vi "Update Value.vi"(6 "Time":dbl, 8 "error in (no error)":errorcluster, 11 "DblPopupControl in":refnum<class "DblPopupControl.lvclass">) -> (0 "error out":errorcluster, 1 "Update":bool, 2 "Value":variant, 3 "DblPopupControl out":refnum<class "DblPopupControl.lvclass">)   [LabVIEW 2020, in "VolatusGUIElements.lvlib" / "DblPopupControl.lvclass"]
uses:
  DblPopupControl.lvclass
  DblPopupControl.lvclass/DblPopupControl.ctl
  lv-vecto/Vecto/Channel DBL/Channel DBL.lvclass/Channel DBL.ctl
  lv-vecto/Vecto/Group DBL/Value by Index.vi
  lv-vecto/Vecto/Channel DBL/Channel DBL.lvclass
  VolatusGUIElements.lvlib
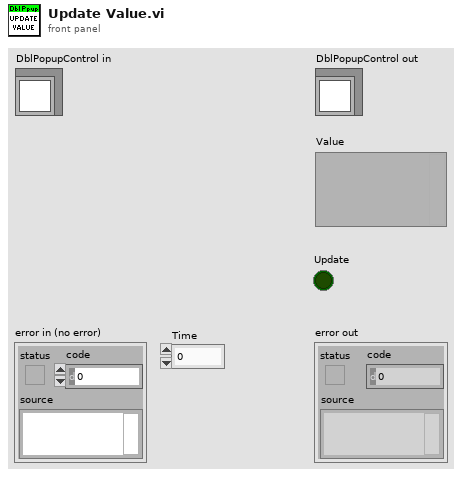
[diagram p1: front panel]
types:
  T1 = typedef "VolatusGUIElements.lvlib/DblPopupControl.lvclass/Cmd State.ctl" = cluster{"Commanding":bool, "Start":dbl, "Error":bool, "Value":dbl}
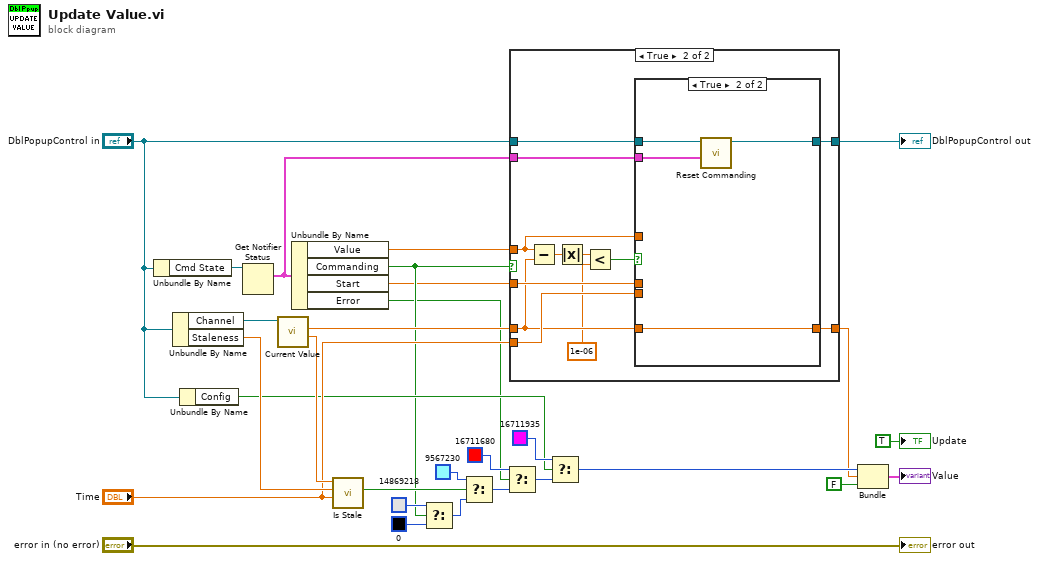
[diagram p0: block diagram]
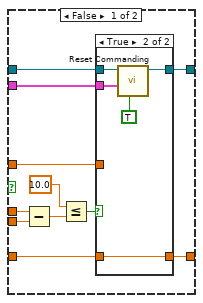
[diagram p3: hidden frame]
diagram:
  n1 = Unbundle By Name("DblPopupControl in") -> ("Cmd State"=w6:refnum<notifier>)
  n2 = Unbundle By Name("DblPopupControl in") -> ("Channel"=w28:refnum<class "Channel DBL.lvclass">, "Staleness"=w26:dbl)
  n3 = Unbundle By Name("DblPopupControl in") -> ("Config"=w11:bool)
  n4 = Get Notifier Status(notifier=w6) -> (current notification=w1:T1)  [unwired: 1 in, 4 out]
  n5 = call "Current Value.vi"("Channel in"=w28) -> ("Timestamp"=w27:dbl, "Scaled"=w16:dbl)  [unwired: 6 in, 3 out]
  n6 = Unbundle By Name(w1) -> ("Value"=w5:dbl, "Commanding"=w4:bool, "Start"=w3:dbl, "Error"=w2:bool)
  n7 = call "Is Stale.vi"("Time"="Time", "Staleness"=w26, "Timestamp"=w27) -> ("Stale"=w20:bool)  [unwired: 8 in]
  n8 = Select(t=u32 14869218, s=w4, f=u32 0) -> (s? t:f=w10:u32)
  n9 = Select(t=u32 9567230, s=w20, f=w10) -> (s? t:f=w24:u32)
  n10 = Select(t=u32 16711680, s=w2, f=w24) -> (s? t:f=w22:u32)
  n11 = case shown="True" w4 {
    tunnel: w16 -> [w31 w41]
    tunnel: w3 -> [_ w43]
    tunnel: "Time" -> [_ w42]
    tunnel: w5 -> [_ w37]
    tunnel: "DblPopupControl in" -> [w30 w40]
    tunnel: [w30 w39] -> w14
    tunnel: [w31 w38] -> w13
    tunnel: w1 -> [_ w32]
    frame False {
    }
    frame True {
      n12 = Subtract(x=w37, y=w41) -> (x-y=w36:dbl)
      n13 = Absolute Value(x=w36) -> (abs(x)=w35:dbl)
      n14 = Less?(x=w35, y=1e-06) -> (x < y?=w33:bool)
      n15 = case shown="True" w33 {
        tunnel: w43 -> [w54 _]
        tunnel: w42 -> [w53 _]
        tunnel: w41 -> [w47 w64]
        tunnel: w40 -> [w49 w65]
        tunnel: [w48 w63] -> w39
        tunnel: [w45 w64] -> w38
        tunnel: w37 -> [w46 _]
        tunnel: w32 -> [w44 w62]
        frame False {
          n16 = Subtract(x=w54, y=w53) -> (x-y=w52:dbl)
          n17 = Less Or Equal?(x=10.0, y=w52) -> (x <= y?=w50:bool)
          n18 = case shown="True" w50 {
            tunnel: w49 -> [w55 w60]
            tunnel: [w55 w59] -> w48
            tunnel: w47 -> [_ w61]
            tunnel: w46 -> [w56 _]
            tunnel: [w56 w61] -> w45
            tunnel: w44 -> [_ w58]
            frame False {
            }
            frame True {
              n19 = call "Reset Commanding.vi"("Error (F)"=TRUE, "Cmd State"=w58, "DblPopupControl in"=w60) -> ("DblPopupControl out"=w59:refnum<class "DblPopupControl.lvclass">)  [unwired: 7 in, 1 out]
            }
          }
        }
        frame True {
          n20 = call "Reset Commanding.vi"("Cmd State"=w62, "DblPopupControl in"=w65) -> ("DblPopupControl out"=w63:refnum<class "DblPopupControl.lvclass">)  [unwired: 8 in, 1 out]
        }
      }
    }
  }
  "DblPopupControl out" <- w14
  n21 = Select(t=u32 16711935, s=w11, f=w22) -> (s? t:f=w19:u32)
  n22 = Bundle(w19, "Scaled"=w13, FALSE) -> (→"Value":cluster{u32, "Scaled":dbl, bool})  [unwired: 1 in]
  "error out" <- "error in (no error)"
  "Update" <- TRUE ("Update")
